vi "create_context_menu.vi"(8 "error in (no error)":errorcluster, 10 "Menus":string[][](array[string]), 11 "BalloonNotifier in":refnum<class "BalloonNotifier.lvclass">) -> (0 "error out":errorcluster, 2 "context menu reference":refnum<k24>, 3 "BalloonNotifier out":refnum<class "BalloonNotifier.lvclass">)   [LabVIEW 2010, in "BalloonNotifier.lvclass"]
uses:
  BalloonNotifier.lvclass
  System.Windows.Forms
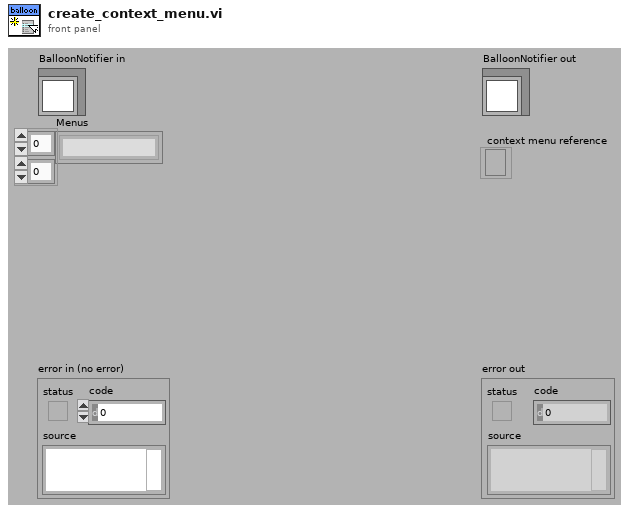
[diagram p1: front panel]
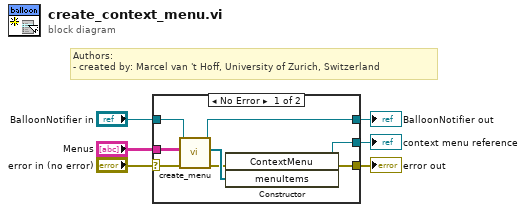
[diagram p0: block diagram]
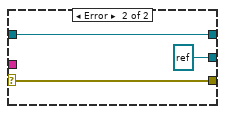
[diagram p2: hidden frame]
diagram:
  # "Authors: \n- created by: Marcel van 't Hoff, University of Zurich, Switzerland"
  n1 = case shown="No Error" "error in (no error)" {
    selector: "error in (no error)" -> [w12 w17]
    tunnel: [w14 w17] -> w5
    tunnel: "Menus" -> [w11 _]
    tunnel: "BalloonNotifier in" -> [w8 w16]
    tunnel: [w7 w16] -> w2
    tunnel: [w13 refnum<k24> refnum ("new reference")] -> w1
    frame No Error {
      n2 = call-dynamic "create_menu.vi"("error in (no error)"=w12, "Menus"=w11, "BalloonNotifier in"=w8) -> ("error out"=w9:errorcluster, "MenuItem references"=w10:refnum<k24>[], "BalloonNotifier out"=w7:refnum<class "BalloonNotifier.lvclass">)  [unwired: 6 in]
      n3 = constructor class="ContextMenu"(error in=w9, "menuItems"=w10) -> (reference out=w13:refnum<k24>, error out=w14:errorcluster)  [unwired: 2 in, 2 out]
    }
    frame Error {
    }
  }
  "error out" <- w5
  "BalloonNotifier out" <- w2
  "context menu reference" <- w1
